vi "Setup.vi"(8 "error in (no error)":errorcluster caption="Fehler (Eingang, kein Fehler)", 11 "Data":T1={"Report.lvclass"=refnum, "test"="", "last State"=enum."do Test", "test ID"=0, "parameter"=[], "EMTestCWS500N.lvclass"=refnum, "CEG4500.lvclass"=refnum, "Tektronix RSA5106A.lvclass"=refnum, "erfolgreich"=FALSE, "log"="", "Kommentar"="", "Device Enum"=enum."unbekannt", "Test Enum"=enum."unbekannt", "debug"=FALSE}) -> (0 "error out":errorcluster, 3 "output cluster":T1={"Report.lvclass"=refnum, "test"="", "last State"=enum."Initialize", "test ID"=0, "parameter"=[], "EMTestCWS500N.lvclass"=refnum, "CEG4500.lvclass"=refnum, "Tektronix RSA5106A.lvclass"=refnum, "erfolgreich"=FALSE, "log"="", "Kommentar"="", "Device Enum"=enum."emTestCWS500N", "Test Enum"=enum."HF-Felder", "debug"=FALSE})   [LabVIEW 2013]
uses:
  Main/controls/Data.ctl
  classes/Datastructure/Report/Report.lvclass
  classes/Devices/emTestCWS500N/EMTestCWS500N.lvclass
  classes/Devices/CEG4500/CEG4500.lvclass
  classes/Devices/Tektronix RSA5106A/Tektronix RSA5106A.lvclass
  Main/controls/State.ctl
  classes/Devices/DeviceInterface/Devices.ctl
  classes/Tests/TestInterface/Tests.ctl
panel:
  out "Tektronix RSA5106A":refnum<visa-resource-name>
  out "CEG 4500":refnum<visa-resource-name>="COM7"
  out "emTestCWS500N1":refnum<visa-resource-name>="COM5"
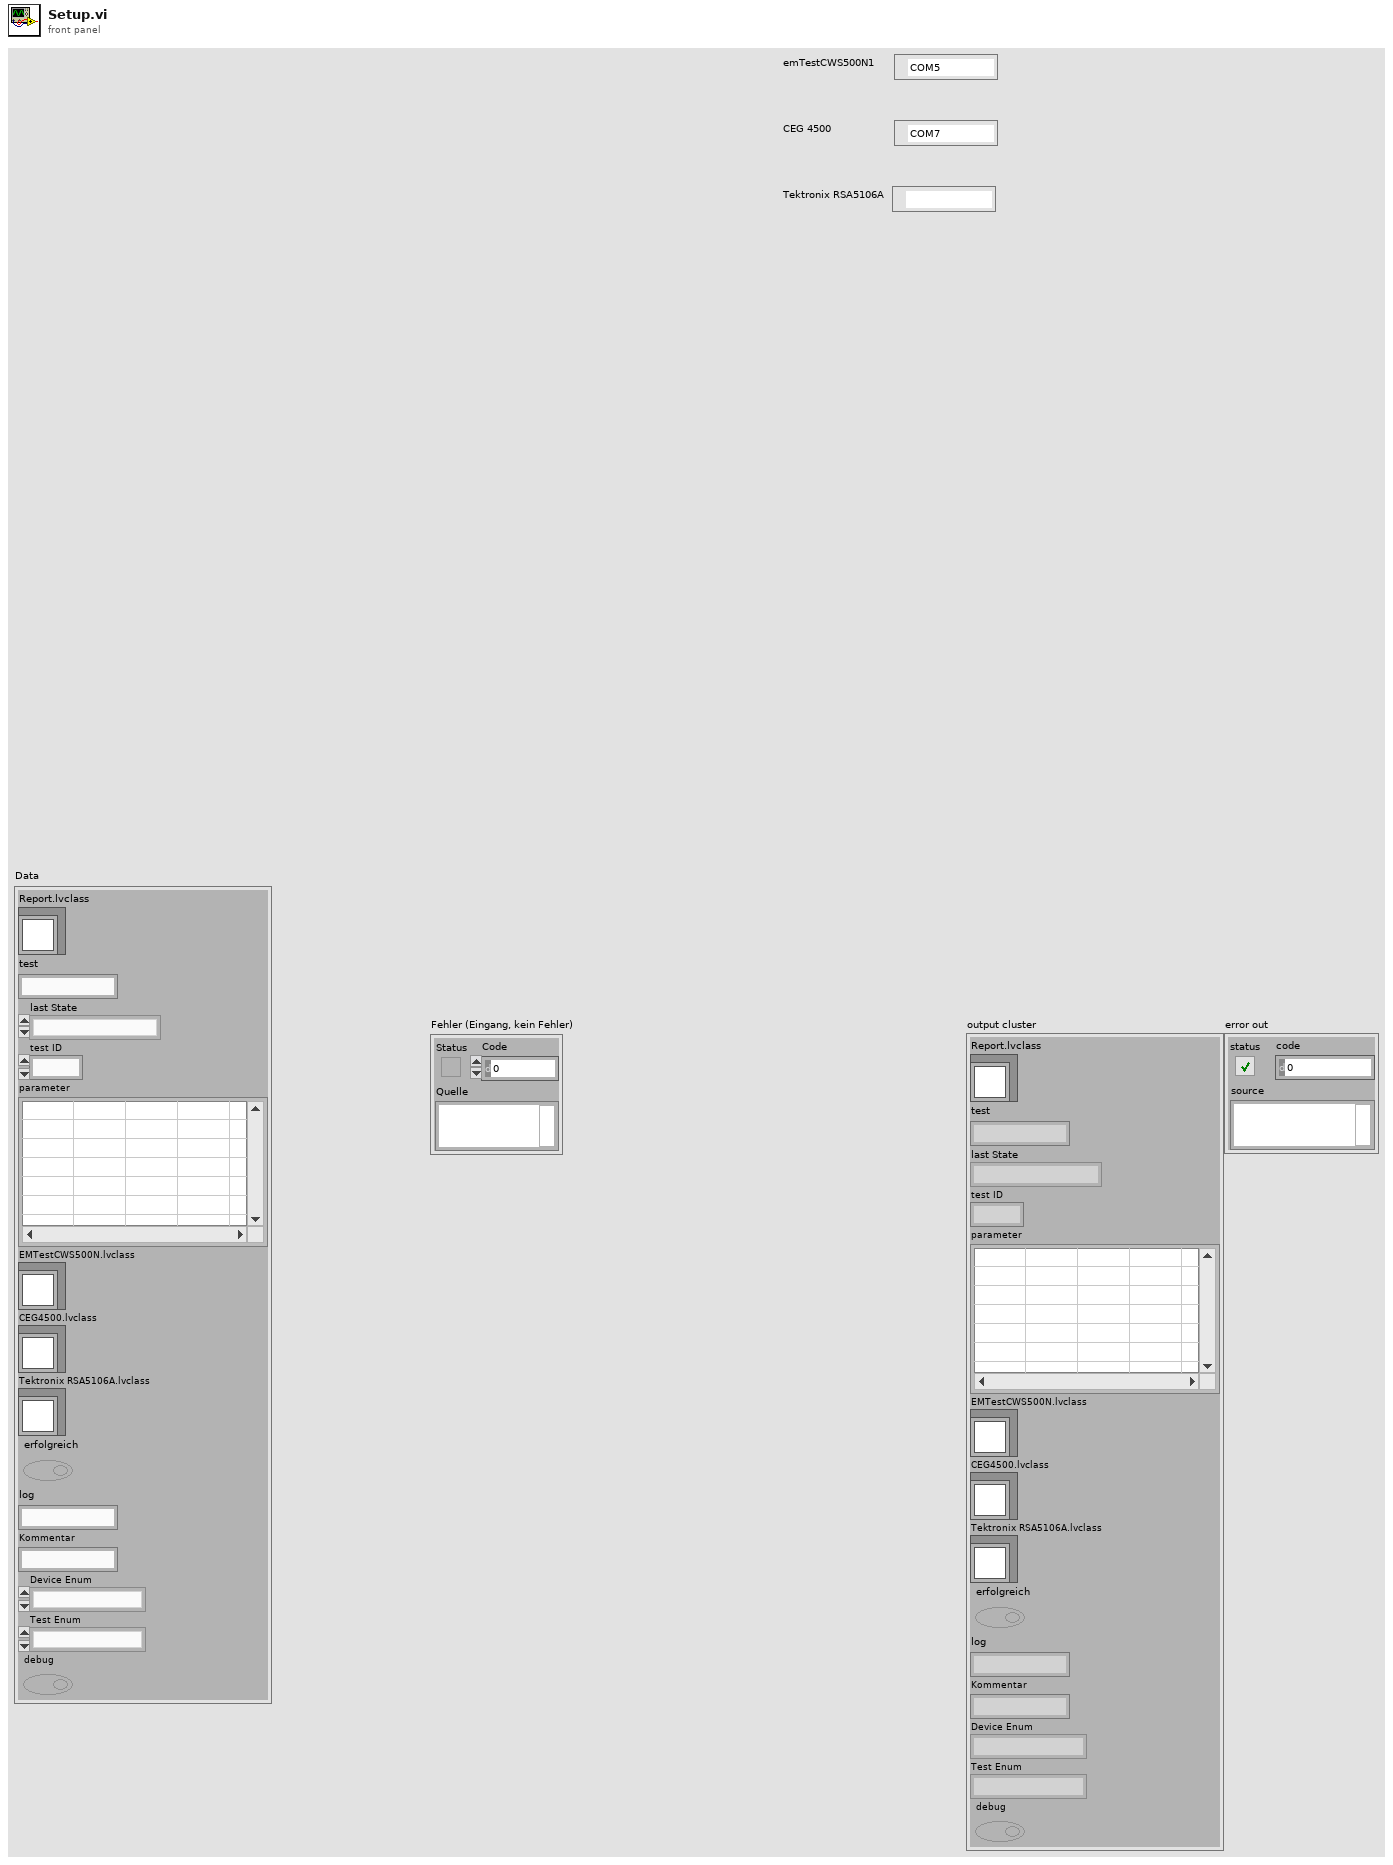
[diagram p1: front panel]
types:
  T1 = typedef "Data.ctl" = cluster{"Report.lvclass":refnum<class "Report.lvclass">, "test":string, "last State":T2, "test ID":i32, "parameter":string[][], "EMTestCWS500N.lvclass":refnum<class "EMTestCWS500N.lvclass">, "CEG4500.lvclass":refnum<class "CEG4500.lvclass">, "Tektronix RSA5106A.lvclass":refnum<class "Tektronix RSA5106A.lvclass">, "erfolgreich":bool, "log":string, "Kommentar":string, "Device Enum":T3, "Test Enum":T4, "debug":bool}
  T2 = typedef "State.ctl" = enum16{"create Pdf", "load Report", "save Report", "do Test", "CDN Kalibrierung", "enter Report Parameters", "new Test", "Protokoll", "read Tree", "update Tree", "Fehler", "Initialize", "Wait for Event", "Exit"}
  T3 = typedef "Devices.ctl" = enum16{"unbekannt", "Tektronix RSA5106A", "emTestCWS500N", "CEG-4500"}
  T4 = typedef "Tests.ctl" = enum16{"unbekannt", "Störaussendung", "Burst", "ESD", "Surge", "Spannungseinbruch", "HF-Felder"}
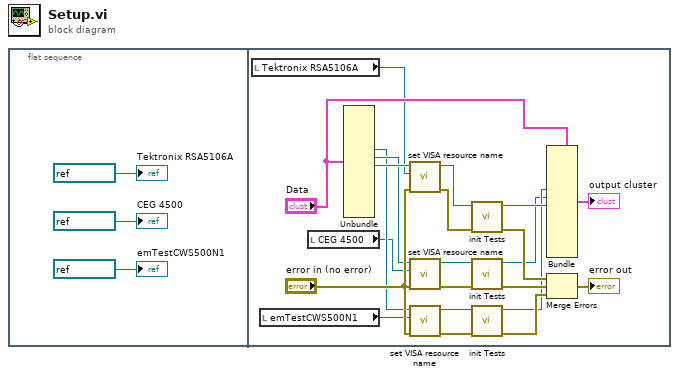
[diagram p0: block diagram]
diagram:
  n1 = flat-sequence {
    frame #0 {
      "emTestCWS500N1" <- refnum<visa-resource-name> "COM5" ("emTestCWS500N1")
      "CEG 4500" <- refnum<visa-resource-name> "COM7" ("CEG 4500")
      "Tektronix RSA5106A" <- refnum<visa-resource-name> "COM4" ("Tektronix RSA5106A")
    }
    frame #1 {
      n2 = local read "Tektronix RSA5106A"() -> (w6:refnum<visa-resource-name>)
      n3 = local read "emTestCWS500N1"() -> (w4:refnum<visa-resource-name>)
      n4 = local read "CEG 4500"() -> (w5:refnum<visa-resource-name>)
      n5 = Unbundle("Data") -> ("EMTestCWS500N.lvclass"=w16:refnum<class "EMTestCWS500N.lvclass">, "CEG4500.lvclass"=w17:refnum<class "CEG4500.lvclass">, "Tektronix RSA5106A.lvclass"=w18:refnum<class "Tektronix RSA5106A.lvclass">)  [unwired: 11 out]
      n6 = call-dynamic "set VISA resource name.vi"("error in (no error)"="error in (no error)", "VISA resource name"=w6, "DeviceInterface (Eingang)"=w18) -> ("error out"=w14:errorcluster, "DeviceInterface (Ausgang)"=w15:refnum<class "Tektronix RSA5106A.lvclass">)  [unwired: 7 in]
      n7 = call-dynamic "set VISA resource name.vi"("error in (no error)"="error in (no error)", "VISA resource name"=w5, "DeviceInterface (Eingang)"=w17) -> ("error out"=w8:errorcluster, "DeviceInterface (Ausgang)"=w9:refnum<class "CEG4500.lvclass">)  [unwired: 7 in]
      n8 = call-dynamic "set VISA resource name.vi"("error in (no error)"="error in (no error)", "VISA resource name"=w4, "DeviceInterface (Eingang)"=w16) -> ("error out"=w11:errorcluster, "DeviceInterface (Ausgang)"=w12:refnum<class "EMTestCWS500N.lvclass">)  [unwired: 7 in]
      n9 = call-dynamic "init Tests.vi"("error in (no error)"=w14, "Tektronix RSA5106A Eingang"=w15) -> ("error out"=w22:errorcluster, "Tektronix RSA5106A Ausgang"=w13:refnum<class "Tektronix RSA5106A.lvclass">)  [unwired: 8 in]
      n10 = call-dynamic "init Tests.vi"("error in (no error)"=w8, "CEG4500 Eingang"=w9) -> ("error out"=w23:errorcluster, "CEG4500 Ausgang"=w7:refnum<class "CEG4500.lvclass">)  [unwired: 8 in]
      n11 = call-dynamic "init Tests.vi"("error in (no error)"=w11, "EMTestCWS500N Eingang"=w12) -> ("error out"=w25:errorcluster, "EMTestCWS500N Ausgang"=w10:refnum<class "EMTestCWS500N.lvclass">)  [unwired: 8 in]
      n12 = Bundle(cluster="Data", "EMTestCWS500N.lvclass"=w10, "CEG4500.lvclass"=w7, "Tektronix RSA5106A.lvclass"=w13) -> (→"output cluster":T1)  [unwired: 11 in]
      n13 = Merge Errors(w22, w23, w25) -> (→"error out":errorcluster)
    }
  }
